vi "Pre Launch Init.vi"(11 "Chat Window in":refnum<class "Chat Window.lvclass">) -> (0 "error out":errorcluster, 3 "Chat Window out":refnum<class "Chat Window.lvclass">)   [LabVIEW 2020, in "Chat Window.lvlib" / "Chat Window.lvclass"]
doc: "(<B>Filename</B>: Actor Framework.lvlib:Actor.lvclass:Pre Launch Init.vi)\n\nDefines behavior that occurs after the Launch Nested Actor method is invoked but before the actor's Actor Core method begins running.\n\nBy default, this method does nothing. A descendant class may override it to define behavior."
uses:
  Chat Window.lvclass
  Chat Window.lvclass/Chat Window.ctl
  <vilib>/ActorFramework/Actor/Actor.lvclass
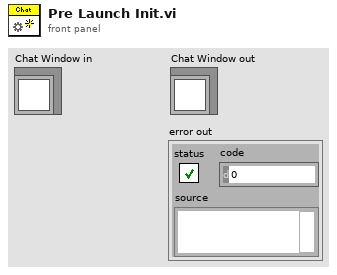
[diagram p1: front panel]
types:
  T1 = cluster{"Stop":refnum<user-event>, "Text":refnum<user-event>, "Connected":refnum<user-event>}
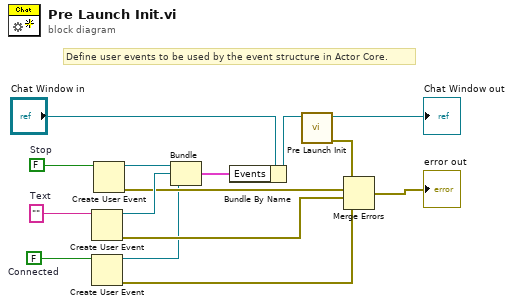
[diagram p0: block diagram]
diagram:
  w3 = FALSE  # Connected
  w12 = FALSE  # Stop
  w13 = ""  # Text
  # "Define user events to be used by the event structure in Actor Core."
  n1 = Create User Event(user event datatype=w13) -> (user event=w10:refnum<user-event>, error out=w6:errorcluster)  [unwired: 1 in]
  n2 = Create User Event(user event datatype=w3) -> (user event=w1:refnum<user-event>, error out=w2:errorcluster)  [unwired: 1 in]
  n3 = Create User Event(user event datatype=w12) -> (user event=w11:refnum<user-event>, error out=w7:errorcluster)  [unwired: 1 in]
  n4 = Bundle("Stop"=w11, "Text"=w10, "Connected"=w1) -> (w8:T1)  [unwired: 1 in]
  n5 = Bundle By Name(cluster="Chat Window in", "Events"=w8) -> (w9:refnum<class "Chat Window.lvclass">)
  n6 = call-parent "Pre Launch Init.vi"("Actor in"=w9) -> ("error out"=w5:errorcluster, "Actor out"=→"Chat Window out":refnum<class "Chat Window.lvclass">)  [unwired: 9 in]
  n7 = Merge Errors(w5, w7, w6, w2) -> (→"error out":errorcluster)
